vi "Calculate Counter And Protections Main Outgoing.vi"(0 "Frames in":T3[](array[typedef]) {"Protection Configurations"."CRC Channels"."Data Type" items=["Signed", "Unsigned", "IEEE Float"]}, 1 "Frame Count":i32, 5 "Protections":T2, 7 "Signals":T1, 9 "Overrides":T1, 11 "error in (no error)":errorcluster, 12 "timeout ms":i32) -> (4 "Frames out":T3[](array[typedef]) {"Protection Configurations"."CRC Channels"."Data Type" items=["Signed", "Unsigned", "IEEE Float"]}, 6 "Frames":T10[](array[typedef]) {"payload" format="%x"; "timestamp" format="%<%.7X\n%x>T"; "type" items=["CAN Data"=0, "CAN Remote"=1, "CAN Bus Error"=2, "CAN 2.0 Data"=8, "CAN FD Data"=16, "CAN FD+BRS Data"=24, "J1939 Data"=192, "Delay"=224, "Log Trigger"=225, "Start Trigger"=226]; "identifier" format="%x"}, 10 "Tick Count(uSec)":u32, 15 "error out":errorcluster)   [LabVIEW 2024, in "Protection and Counter Support Engine.lvlib"]
uses:
  Protection and Counter Support Engine.lvlib
  <vilib>/xnet/xnet.llb/XNET Frame CAN.ctl
  <vilib>/xnet/xnet.llb/XNET Frame Type CAN.ctl
  Types/RT Frame Settings.ctl
  Shared/Types/Exported Frame Type.ctl
  Types/RT Protection Configuration.ctl
  Shared/Types/Protection Type.ctl
  Shared/Types/XNET Signal Configuration.ctl
  Shared/Types/Exported Counter Settings.ctl
  Shared/Types/Exported Event Trigger Type.ctl
  <vilib>/NI/NIVS Inline Async API/_Data Access Engine/Data Access Engine/Types/Read.DVR.ctl
  <vilib>/NI/NIVS Inline Async API/_Data Access Engine/Access Type Classes/Read/Read.lvclass
  <vilib>/NI/NIVS Inline Async API/_Data Access Engine/Data Access Engine/Types/Write.DVR.ctl
  <vilib>/NI/NIVS Inline Async API/_Data Access Engine/Access Type Classes/Write/Write.lvclass
  <vilib>/NI/NIVS Inline Async API/_Data Access Engine/Access Type Classes/Read/Read.lvclass/Read.ctl
  <vilib>/NI/NIVS Inline Async API/_Data Access Engine/Access Type Classes/Write/Write.lvclass/Write.ctl
  <vilib>/NI/NIVS Inline Async API/_Data Access Engine/Data Access Engine/Methods/Write.Data.Commit.vi
  <vilib>/NI/NIVS Inline Async API/_Data Access Engine/Data Access Engine/Methods/Read.Data.Detect.vi
  <vilib>/NI/NIVS Inline Async API/_Data Access Engine/Data Access Engine/Methods/Read.Data.vi
  Determine Transmission.vi
  Determine Periodic.vi
  Set Counter Signal.vi
  Calculate Counter Value.vi
  Set Protection Signal.vi
  Calculate Protection Value.vi
  <vilib>/NI/NIVS Inline Async API/_Data Access Engine/Access Type Classes/Write/Write.Commit.vi
  <vilib>/NI/NIVS Inline Async API/_Data Access Engine/Access Type Classes/Read/Read.ProcessData.Detect.vi
  <vilib>/NI/NIVS Inline Async API/_Data Access Engine/Access Type Classes/Read/Read.ProcessData.vi
  <vilib>/NI/NIVS Inline Async API/_Data Access Engine/Data Access Engine/Methods/Write.Data.Buffer.vi
  Get Protection Signals.vi
  <vilib>/NI/NIVS Inline Async API/_Data Access Engine/Access Type Classes/Write/Write.Buffer.vi
  <vilib>/xnet/xnet.llb/XNET Convert.vi
  <vilib>/xnet/xnet.llb/XNET Convert (Signal to Frame Raw).vi
  <vilib>/xnet/xnet.llb/XNET Convert (Signal to Frame CAN).vi
  <vilib>/NI/NIVS Inline Async API/_Data Access Engine/Data Access Engine/Data Access Engine.lvclass
  Shared/Protection and Counter Support Shared.lvlib
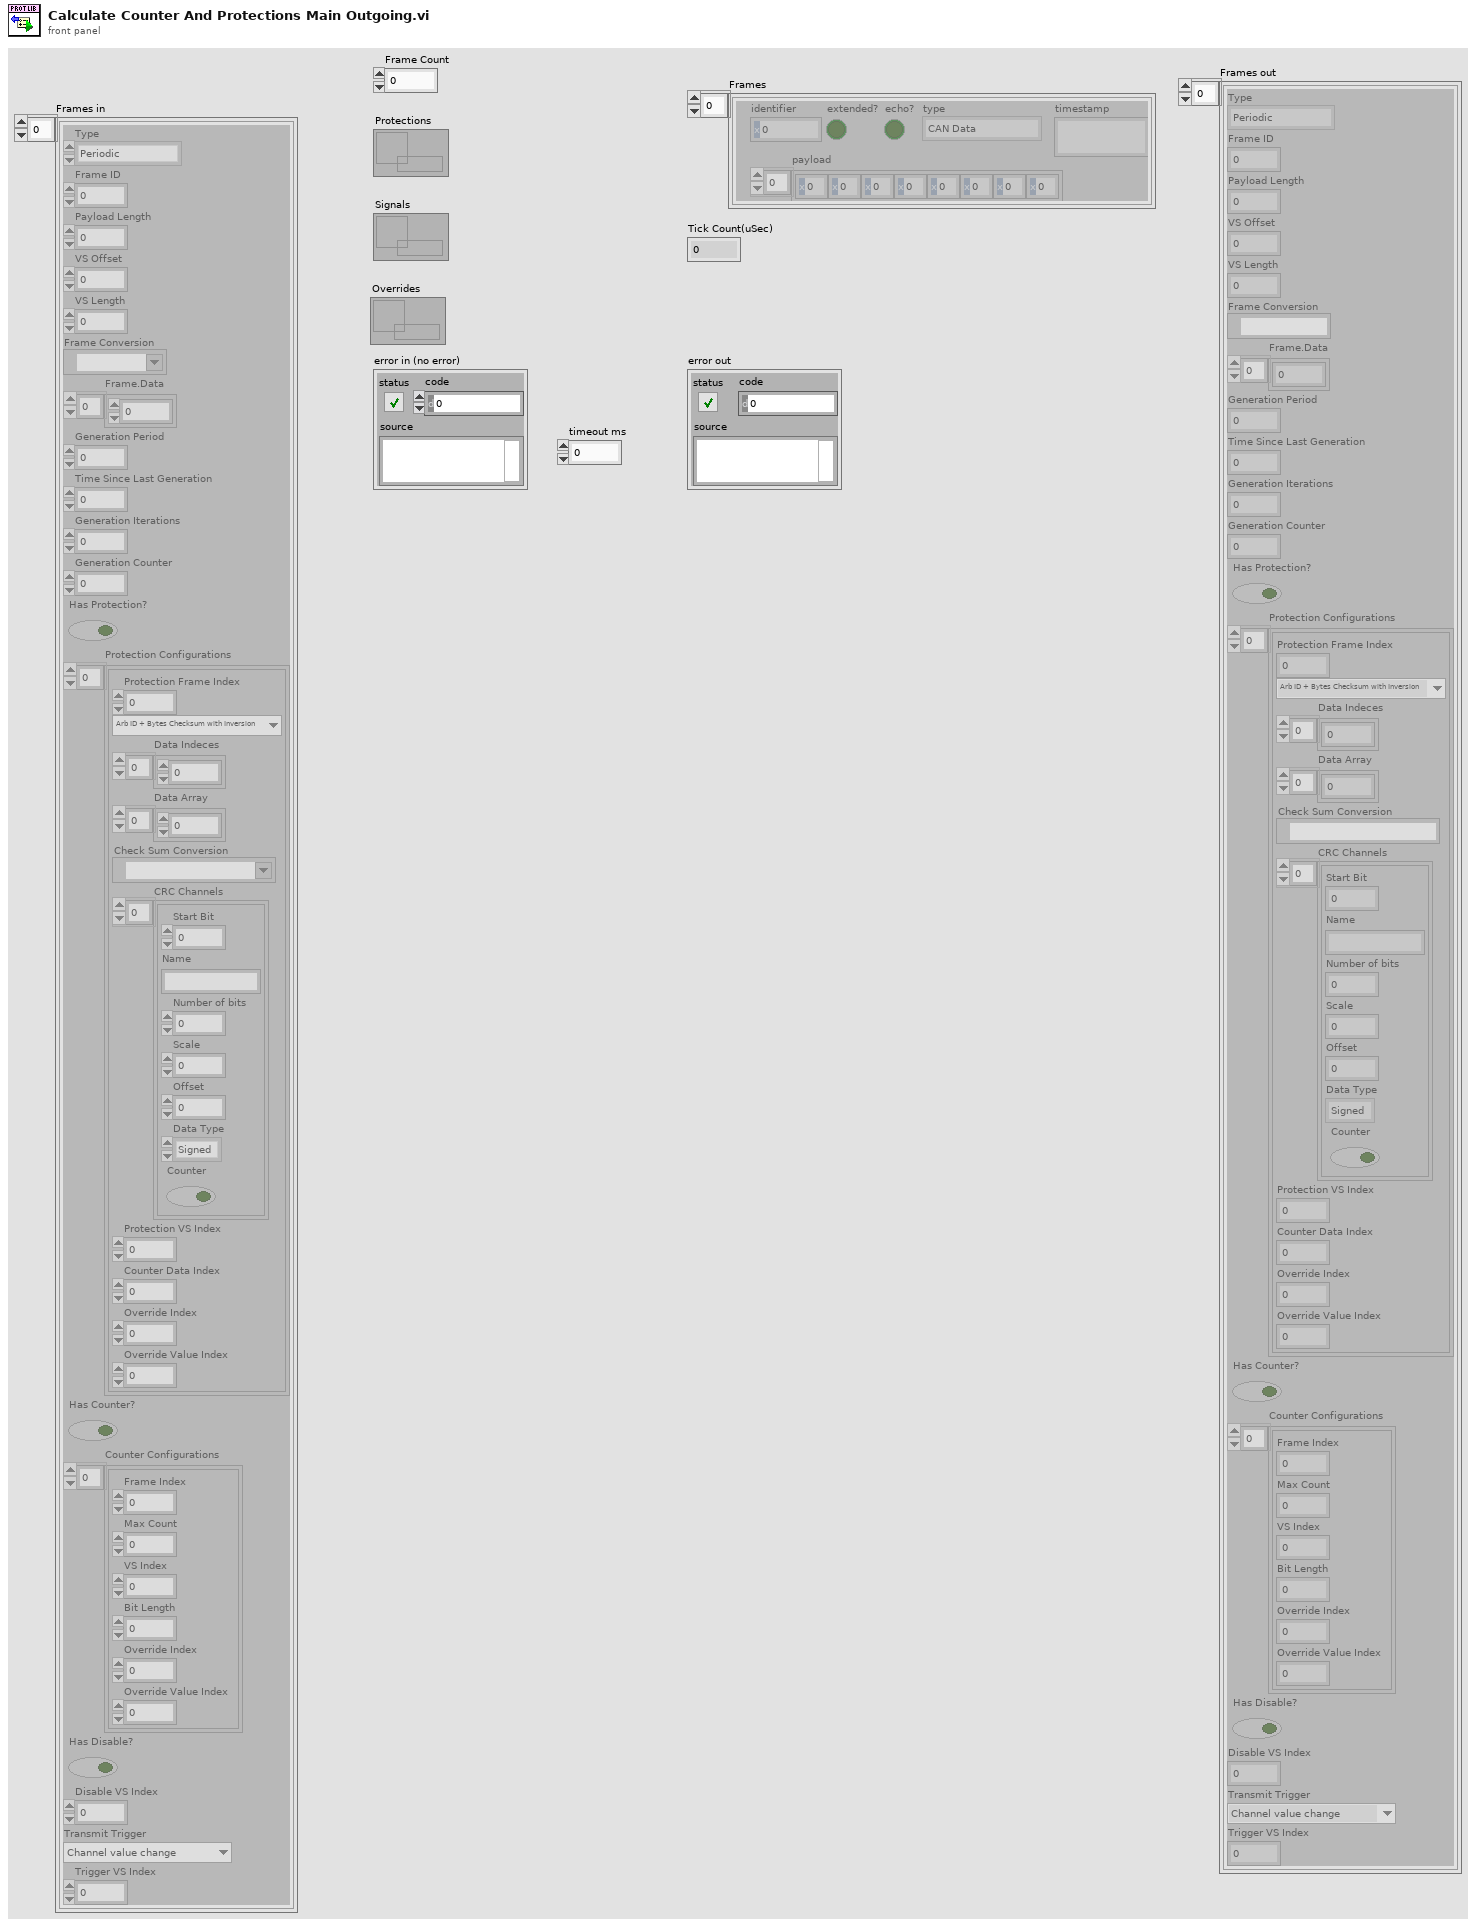
[diagram p1: front panel]
types:
  T1 = typedef "Data Access Engine.lvlib/Data Access Engine.lvclass/Read.DVR.ctl" = refnum<data-value>
  T2 = typedef "Data Access Engine.lvlib/Data Access Engine.lvclass/Write.DVR.ctl" = refnum<data-value>
  T3 = typedef "Protection and Counter Support Engine.lvlib/RT Frame Settings.ctl" = cluster{"Type":T4, "Frame ID":u32, "Payload Length":u32, "VS Offset":i32, "VS Length":i32, "Frame Conversion":refnum<k21>, "Frame.Data":dbl[], "Generation Period":u32, "Time Since Last Generation":u32, "Generation Iterations":u32, "Generation Counter":u32, "Has Protection?":bool, "Protection Configurations":T5[], "Has Counter?":bool, "Counter Configurations":T8[], "Has Disable?":bool, "Disable VS Index":i32, "Transmit Trigger":T9, "Trigger VS Index":i32}
  T4 = typedef "Protection and Counter Support Shared.lvlib/Exported Frame Type.ctl" = enum16{"Periodic", "Event", "Periodic/Event"}
  T5 = typedef "Protection and Counter Support Engine.lvlib/RT Protection Configuration.ctl" = cluster{"Protection Frame Index":i32, "Protection Type":T6, "Data Indeces":i32[], "Data Array":dbl[], "Check Sum Conversion":refnum<k21>, "CRC Channels":T7[], "Protection VS Index":i32, "Counter Data Index":i32, "Override Index":i32, "Override Value Index":i32}
  T6 = typedef "Protection and Counter Support Shared.lvlib/Protection Type.ctl" = enum16{"Arb ID + Bytes Checksum with Inversion", "Arb ID + Bytes CRC with Inversion", "Reversed Raw Signal Checksum with Inversion", "Concatenated Two's Compliment"}
  T7 = typedef "Protection and Counter Support Shared.lvlib/XNET Signal Configuration.ctl" = cluster{"Start Bit":i32, "Name":string, "Number of bits":i32, "Scale":dbl, "Offset":dbl, "Data Type":u32, "Counter":bool}
  T8 = typedef "Protection and Counter Support Shared.lvlib/Exported Counter Settings.ctl" = cluster{"Frame Index":i32, "Max Count":dbl, "VS Index":i32, "Bit Length":i64, "Override Index":i32, "Override Value Index":i32}
  T9 = typedef "Protection and Counter Support Shared.lvlib/Exported Event Trigger Type.ctl" = enum16{"Channel value change", "Trigger channel (not zero)", "Channel value change or trigger channel (not zero)", "Trigger channel (any value change)", "Channel value change or trigger channel (any value change)"}
  T10 = typedef "XNET Frame CAN.ctl" = cluster{"timestamp":timestamp, "payload":u8[], "identifier":u32, "type":T11, "extended?":bool, "echo?":bool}
  T11 = typedef "XNET Frame Type CAN.ctl" = u8
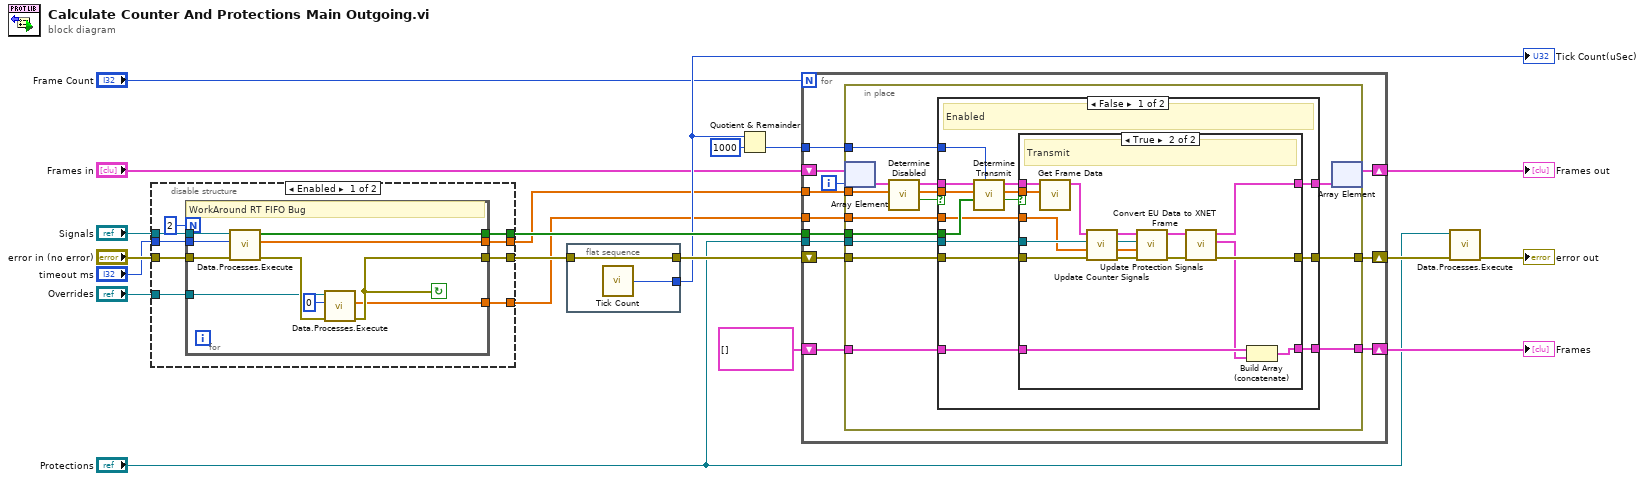
[diagram p0: block diagram]
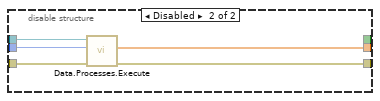
[diagram p2: hidden frame]
diagram:
  n1 = disable-structure shown="Enabled" {
    disable-tunnel: "timeout ms" -> [w29 w44]
    disable-tunnel: [w28 w43] -> w19
    disable-tunnel: [w27 w42] -> w5
    disable-tunnel: "error in (no error)" -> [w26 w41]
    disable-tunnel: "Signals" -> [w25 w40]
    disable-tunnel: [w23 _] -> w11
    disable-tunnel: [w22 _] -> w2
    disable-tunnel: "Overrides" -> [w21 _]
    frame Enabled {
      n2 = for {
        N: 2 -> [_]
        tunnel: w29 -> [w39]
        tunnel: [w38] -> w27
        tunnel: w25 -> [w36]
        tunnel: w26 -> [w37]
        tunnel: [w33] -> w28
        tunnel: [w35] -> w23
        tunnel: [w31] -> w22
        tunnel: w21 -> [w30]
        stop <- w33 continue-if-true
        # "WorkAround RT FIFO Bug"
        n3 = call-poly <vilib>:"Data.Processes.Execute.vi"("error in (no error)"=w37, "timeout ms"=w39, "Ref"=w36) -> ("error out"=w34:errorcluster, "Values"=w38:dbl[], "Detect?"=w35:bool[])  [unwired: 5 in, 1 out]
        n4 = call-poly <vilib>:"Data.Processes.Execute.vi"("error in (no error)"=w34, "timeout ms"=0, "Ref"=w30) -> ("error out"=w33:errorcluster, "Values"=w31:dbl[])  [unwired: 6 in, 1 out]
      }
    }
    frame Disabled {
      n5 = call-poly <vilib>:"Data.Processes.Execute.vi"("error in (no error)"=w41, "timeout ms"=w44, "Ref"=w40) -> ("error out"=w43:errorcluster, "Values"=w42:dbl[])  [unwired: 6 in, 1 out]
    }
  }
  n6 = flat-sequence {
    tunnel: [w46] -> w10
    tunnel: [w45] -> w20
    tunnel: w19 -> [w45]
    frame #0 {
      n7 = call "Tick Count"() -> ("Tick Count(uSec)"=w46:u32)
    }
  }
  n8 = Quotient & Remainder(x=w10, y=u32 1000) -> (floor(x/y)=w13:u32)  [unwired: 1 out]
  n9 = for {
    N: "Frame Count" -> [_]
    tunnel: w5 -> [w55]
    shift-right: [w57] -> w17
    shift-left: w20 -> [w58]
    tunnel: w13 -> [w56]
    tunnel: "Protections" -> [w54]
    shift-right: [w51] -> w12
    shift-left: "Frames in" -> [w53]
    tunnel: w11 -> [w50]
    shift-right: [w49] -> w16
    shift-left: T10[] [] -> [w48]
    tunnel: w2 -> [w47]
    i -> [w52]
    n10 = in-place {
      in-place-border: w58 -> [w72]
      in-place-border: [w71] -> w57
      in-place-border: w56 -> [w70]
      in-place-border: w55 -> [w69]
      in-place-border: w54 -> [w68]
      in-place-border: w50 -> [w67]
      in-place-border: [w66] -> w49
      in-place-border: w48 -> [w65]
      in-place-border: w47 -> [w59]
      n11 = in-place-array #1(w53, w52) -> (w64:T3)
      n12 = call "Determine Disabled.vi"("Values in"=w69, "Frame Settings in"=w64) -> ("Disabled?"=w61:bool, "Values out"=w60:dbl[], "Frame Settings out"=w63:T3)  [unwired: 7 in]
      n13 = case shown="False" w61 {
        tunnel: w72 -> [w85 w109]
        tunnel: [w86 w109] -> w71
        tunnel: w70 -> [w74 _]
        tunnel: w68 -> [w81 _]
        tunnel: w67 -> [w84 _]
        tunnel: [w83 w108] -> w66
        tunnel: w65 -> [w82 w108]
        tunnel: w63 -> [w79 w107]
        tunnel: [w78 w107] -> w62
        tunnel: w60 -> [w77 _]
        tunnel: w59 -> [w73 _]
        frame False {
          # "Enabled"
          n14 = call "Determine Transmit.vi"("Current Time"=w74, "Detect?"=w84, "Values"=w77, "Frame Settings in"=w79) -> ("Transmit"=w76:bool, "Values out"=w75:dbl[], "Frame Settings out"=w80:T3)  [unwired: 5 in]
          n15 = case shown="True" w76 {
            tunnel: [w89 w105] -> w86
            tunnel: w85 -> [w89 w104]
            tunnel: [w88 w95] -> w83
            tunnel: w82 -> [w88 w97]
            tunnel: w81 -> [_ w102]
            tunnel: w80 -> [w87 w101]
            tunnel: [w87 w98] -> w78
            tunnel: w75 -> [_ w92]
            tunnel: w73 -> [_ w91]
            frame False {
              # "Do not transmit"
            }
            frame True {
              # "Transmit"
              n16 = call "Get Frame Data.vi"("Values"=w92, "Frame Settings in"=w101) -> ("Frame Settings out"=w100:T3)  [unwired: 9 in]
              n17 = call "Update Counter Signals.vi"("error in (no error)"=w104, "Overrides"=w91, "Protections"=w102, "Frame Settings in"=w100) -> ("error out"=w103:errorcluster, "Overrides out"=w90:dbl[], "Protections out"=w94:T2, "Frame Settings out"=w93:T3)  [unwired: 4 in]
              n18 = call "Update Protection Signals.vi"("error in (no error)"=w103, "Overrides"=w90, "Protections"=w94, "Frame Settings in"=w93) -> ("error out"=w106:errorcluster, "Frame Settings out"=w99:T3)  [unwired: 6 in]
              n19 = call "Convert EU Data to XNET Frame.vi"("error in (no error)"=w106, "Frame Settings in"=w99) -> ("error out"=w105:errorcluster, "Frames List"=w96:T10[], "Frame Settings out"=w98:T3)  [unwired: 7 in]
              n20 = Build Array (concatenate)(w97, w96) -> (w95:T10[])
            }
          }
        }
        frame True {
          # "Disabled"
        }
      }
      n21 = in-place-array #1(w62) -> (w51:T3[])  [unwired: 1 out]
    }
  }
  "Frames" <- w16
  "Frames out" <- w12
  n22 = call-poly <vilib>:"Data.Processes.Execute.vi"("error in (no error)"=w17, "Ref"="Protections") -> ("error out"=→"error out":errorcluster)  [unwired: 9 in]
  "Tick Count(uSec)" <- w10
